vi "4.2 Arguments - Error As Arguments.vi"() -> ()   [LabVIEW 2017]
doc: "### 4.2 Arguments - Error As Arguments.vi\n\n#### Overview\n\nConverts a LabVIEW error cluster into a CSM-compatible error string, which allows the CSM core parse engine to process LabVIEW errors from the message queue. The converted error string uses the following format: `[Error: error-code] error-description-As-safe-argument-string`.\n\n#### Introduction\n\nThis example converts a LabVIEW error cluster into a CSM-compatible error string, which allows the CSM core parse engine to process LabVIEW errors from the message queue. The converted error string uses the following format: `[Error: error-code] error-description-As-safe-argument-string`. Furthermore, the CSM-Argument Type.vi gets the argument token, in this case `ErrStr`."
uses:
  user.lib/_NEVSTOP/Communicable State Machine(CSM)/AdvanceAPI/CSM - Revert Arguments-Safe String.vi
  user.lib/_NEVSTOP/Communicable State Machine(CSM)/AdvanceAPI/CSM - Make String Arguments Safe.vi
  user.lib/_NEVSTOP/Communicable State Machine(CSM)/AdvanceAPI/CSM - Keywords.vi
  user.lib/_NEVSTOP/Communicable State Machine(CSM)/_Shared/Trim Single-line Text.vi
  user.lib/_NEVSTOP/Communicable State Machine(CSM)/Communicable State Machine.lvlib
  user.lib/_NEVSTOP/Communicable State Machine(CSM)/_Shared/CSM Shared.lvlib
panel:
  out "error 2":errorcluster
  out "Warning Arguments":string
  out "argument token":string
  out "<ErrStr>[Error: 472]Error String 1%0AError String 2%0AError String 3":errorcluster
  out "[Error: 502]Error String 1%0AError String 2%0AError String 3":errorcluster
  out "Error Arguments":string
  out "error":errorcluster
  # "#CSM-Example Overview\n\nConverts a LabVIEW error cluster into a CSM-compatible error string, which allows the CSM core parse engine to process LabVIEW errors from the message queue. The converted error string uses the following format: `[Error: error-code] error-description-As-safe-argument-string`."
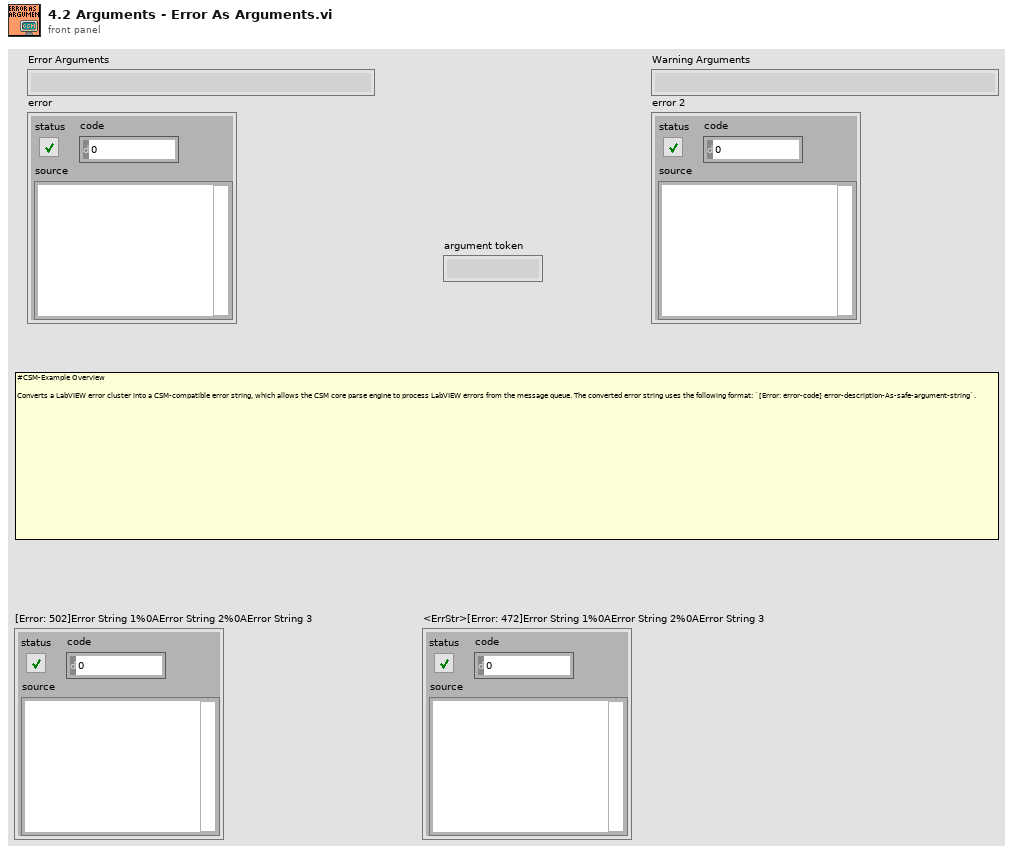
[diagram p1: front panel]
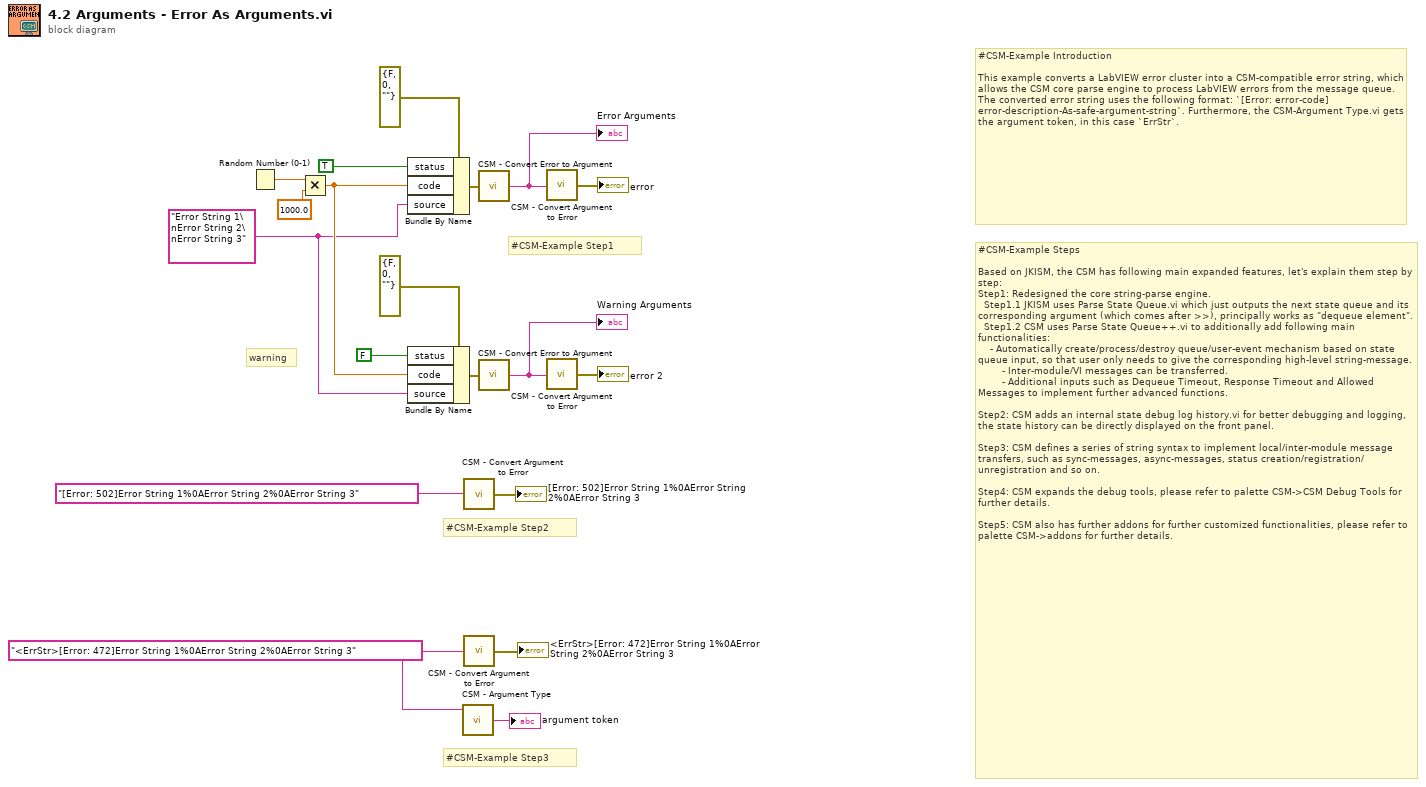
[diagram p0: block diagram]
diagram:
  w9 = "<ErrStr>[Error: 472]Error String 1%0AError String 2%0AError String 3" ("Arguments 2")
  w1 = "Error String 1\nError String 2\nError String 3" ("source")
  # "warning"
  # "#CSM-Example Step3"
  # "#CSM-Example Step2"
  # "#CSM-Example Step1"
  # "#CSM-Example Steps\n\nBased on JKISM, the CSM has following main expanded features, let's explain them step by step:\nStep1: Redesigned the core string-parse engine.\n  Step1.1 JKISM uses Parse State Queue.vi which just outputs the next state queue and its corresponding argument (which comes after >>), principally works as \"dequeue element\".\n  Step1.2 CSM uses Parse State Queue++.vi to additionally add following main functionalities:\n    - Automatically create/process/destroy queue/user-event mechanism based on state queue input, so that user only needs to give the corresponding high-level string-message.\n        - Inter-module/VI messages can be transferred.\n        - Additional inputs such as Dequeue Timeout, Response Timeout and Allowed Messages to implement further advanced functions. \n\nStep2: CSM adds an internal state debug log history.vi for better debugging and logging, the state history can be directly displayed on the front panel.\n\nStep3: CSM defines a series of string syntax to implement local/inter-module message transfers, such as sync-messages, async-messages, status creation/registration/unregistration and so on.\n\nStep4: CSM expands the debug tools, please refer to palette CSM->CSM Debug Tools for further details.\n\nStep5: CSM also has further addons for further customized functionalities, please refer to palette CSM->addons for further details."
  # "#CSM-Example Introduction\n\nThis example converts a LabVIEW error cluster into a CSM-compatible error string, which allows the CSM core parse engine to process LabVIEW errors from the message queue. The converted error string uses the following format: `[Error: error-code] error-description-As-safe-argument-string`. Furthermore, the CSM-Argument Type.vi gets the argument token, in this case `ErrStr`."
  n1 = Random Number (0-1)() -> (number: 0 to 1=w15:dbl)
  n2 = Multiply(x=w15, y=1000.0) -> (x*y=w2:dbl)
  n3 = Bundle By Name(cluster=errorcluster {"status"=FALSE, "code"=0, "source"=""} ("error constant"), "status"=TRUE, "code"=w2, "source"=w1) -> (w17:errorcluster)
  n4 = Bundle By Name(cluster=errorcluster {"status"=FALSE, "code"=0, "source"=""} ("error constant"), "status"=FALSE, "code"=w2, "source"=w1) -> (w5:errorcluster)
  n5 = call "CSM - Argument Type.vi"("Arguments"=w9) -> ("Argument Type"=→"argument token":string)  [unwired: 3 in, 1 out]
  n6 = call "CSM - Convert Argument to Error.vi"("Argument"="[Error: 502]Error String 1%0AError String 2%0AError String 3" ("Arguments 2")) -> ("Error"=→"[Error: 502]Error String 1%0AError String 2%0AError String 3":errorcluster)  [unwired: 4 in]
  n7 = call "CSM - Convert Argument to Error.vi"("Argument"=w9) -> ("Error"=→"<ErrStr>[Error: 472]Error String 1%0AError String 2%0AError String 3":errorcluster)  [unwired: 4 in]
  n8 = call "CSM - Convert Error to Argument.vi"("Error"=w17) -> ("Argument"=w13:string)  [unwired: 4 in]
  "Error Arguments" <- w13
  n9 = call "CSM - Convert Error to Argument.vi"("Error"=w5) -> ("Argument"=w7:string)  [unwired: 4 in]
  "Warning Arguments" <- w7
  n10 = call "CSM - Convert Argument to Error.vi"("Argument"=w13) -> ("Error"=→"error":errorcluster)  [unwired: 4 in]
  n11 = call "CSM - Convert Argument to Error.vi"("Argument"=w7) -> ("Error"=→"error 2":errorcluster)  [unwired: 4 in]
